vi "User_Defined_Test_MinimumJerkGenerateNext.vi"() -> (3 "Unit Test Framework Results":T1)   [LabVIEW 2016]
doc: "Use this template to create a user-defined test VI. Define your test requirements and wire the results to the <b>Result (Test)</b> control. Do not modify the <b>Unit Test Framework Results</b> indicator."
uses:
  <vilib>/utf/common/utf_test_result_troll.ctl
  <vilib>/utf/common/utf_test_result.ctl
  <vilib>/utf/common/utf_test_result_failure.ctl
  <vilib>/utf/common/utf_test_comparison_operators.ctl
  <vilib>/utf/common/utf_vi_tag.ctl
  MyPAM Controller/Controls/timer control.ctl
  MyPAM Controller/Controls/initial conditions control.ctl
  MyPAM Controller/Controls/tf control.ctl
  <vilib>/Control Software Solutions Ltd/UTF Helper/SubVIs/UTF Double Equals.vi
  MyPAM Controller/controllerLibrary.lvlib
  <vilib>/Control Software Solutions Ltd/UTF Helper/Unit Test Helper.lvlib
  <vilib>/utf/NI_UnitTestFramework.lvlib
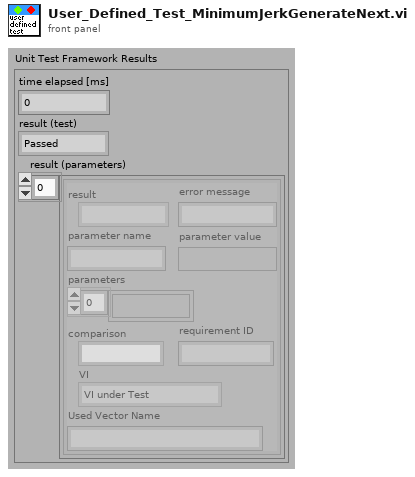
[diagram p1: front panel]
types:
  T1 = typedef "NI_UnitTestFramework.lvlib/utf_test_result_troll.ctl" = cluster{"time elapsed [ms]":u32, "result (test)":T2, "result (parameters)":T3[]}
  T2 = typedef "NI_UnitTestFramework.lvlib/utf_test_result.ctl" = enum16{"Passed", "Failed", "Error", "Skipped", "Not Processed"}
  T3 = typedef "NI_UnitTestFramework.lvlib/utf_test_result_failure.ctl" = cluster{"result":T2, "error message":string, "parameter name":string, "parameter value":variant, "parameters":variant[], "comparison":T4, "requirement ID":string, "VI":T5, "Used Vector Name":string}
  T4 = typedef "NI_UnitTestFramework.lvlib/utf_test_comparison_operators.ctl" = enum16{"=", "!=", ">", ">=", "<", "<=", "range", "symmetric tolerance", "asymmetric tolerance", "string contains", "string not contain", "array size", "string length", "array range", "by element", "array range (limit array)", "user-defined", "array contains", "array not contain", "vector length", "= (elm)", "!= (elm)", "= (case insensitive)", "!= (case insensitive)"}
  T5 = typedef "NI_UnitTestFramework.lvlib/utf_vi_tag.ctl" = enum16{"Setup VI", "VI under Test", "Teardown VI"}
  T6 = typedef "controllerLibrary.lvlib/tf control.ctl" = enum16{"get tf", "set tf"}
  T7 = typedef "controllerLibrary.lvlib/initial conditions control.ctl" = enum16{"get", "set"}
  T8 = typedef "controllerLibrary.lvlib/timer control.ctl" = enum16{"get time", "set time"}
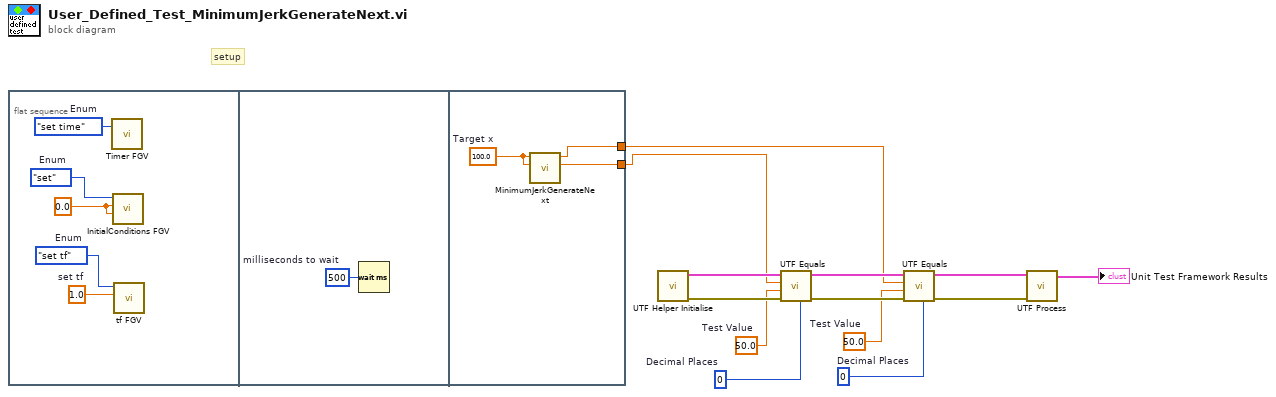
[diagram p0: block diagram]
diagram:
  w1 = u8 0  # Decimal Places
  w2 = u8 0  # Decimal Places
  w5 = 50.0  # Test Value
  w6 = 50.0  # Test Value
  # "setup"
  n1 = flat-sequence {
    tunnel: [w21] -> w4
    tunnel: [w20] -> w3
    frame #0 {
      w14 = 1.0  # set tf
      w15 = tf_control."set tf"  # Enum
      w16 = 0.0 ("X0")
      w17 = initial_conditions_control."set"  # Enum
      w18 = timer_control."set time"  # Enum
      n2 = call "Timer FGV.vi"("Enum"=w18) -> ()  [unwired: 10 in, 1 out]
      n3 = call "InitialConditions FGV.vi"("Y0"=w16, "X0"=w16, "Enum"=w17) -> ()  [unwired: 7 in, 2 out]
      n4 = call "tf FGV.vi"("set tf"=w14, "Enum"=w15) -> ()  [unwired: 9 in, 1 out]
    }
    frame #1 {
      w19 = u32 500  # milliseconds to wait
      n5 = Wait (ms)(milliseconds to wait=w19) -> ()  [unwired: 1 out]
    }
    frame #2 {
      w22 = 100.0  # Target x
      n6 = call "MinimumJerkGenerateNext.vi"("Target y"=w22, "Target x"=w22) -> ("yt"=w20:dbl, "xt"=w21:dbl)  [unwired: 8 in]
    }
  }
  n7 = call <vilib>:"UTF Helper Initialise.vi"() -> ("error out"=w11:errorcluster, "results array"=w12:T3[])  [unwired: 10 in]
  n8 = call-poly <vilib>:"UTF Equals.vi"("Decimal Places"=w2, "error in (no error)"=w11, "Test Value"=w6, "Input"=w3, "Input Results"=w12) -> ("error out"=w9:errorcluster, "Output Results"=w10:T3[])  [unwired: 5 in]
  n9 = call-poly <vilib>:"UTF Equals.vi"("Decimal Places"=w1, "error in (no error)"=w9, "Test Value"=w5, "Input"=w4, "Input Results"=w10) -> ("error out"=w7:errorcluster, "Output Results"=w8:T3[])  [unwired: 5 in]
  n10 = call <vilib>:"UTF Process.vi"("error in (no error)"=w7, "results array"=w8) -> ("Unit Test Framework Results"=→"Unit Test Framework Results":T1)  [unwired: 9 in]
